vi "Find Data Replay Channels.vi"(6 "Custom Device Ref":T2 format="%.0x", 7 "Control String Info":T1, 8 "error in (no error)":errorcluster, 9 "Channel Descriptors in":T3, 11 "Replay ref":T2 format="%.0x") -> (0 "error out":errorcluster, 1 "Channel Descriptors out":T3)   [LabVIEW 2011, in "Engine Sim System Explorer.lvlib"]
uses:
  Engine Sim System Explorer.lvlib
  <vilib>/NI Veristand/Custom Device API/Custom Device Item Ref.ctl
  Shared/Channel Descriptors.ctl
  Shared/FPGA Write Descriptor.ctl
  Shared/InputChannelTypes.ctl
  <vilib>/rvi/DataTransferAndStorage/Container/Common/niFpgaDataTypeControl.ctl
  Shared/FPGA Read Descriptor.ctl
  Shared/OutputChannelTypes.ctl
  Shared/Status Chan Descriptor.ctl
  TypeDefs/DataReplayCtrlStringInfo.ctl
  Shared/Engine Simulation Global.vi
  <vilib>/NI Veristand/Custom Device Tools/Custom Device Utility Library/NI VeriStand - Search for Item by Name.vi
  <vilib>/NI Veristand/Custom Device Tools/Custom Device Utility Library/Custom Device Utility Library.lvlib
  Engine Simulation Shared.lvlib
  <vilib>/NI Veristand/Custom Device API/Custom Device API.lvlib
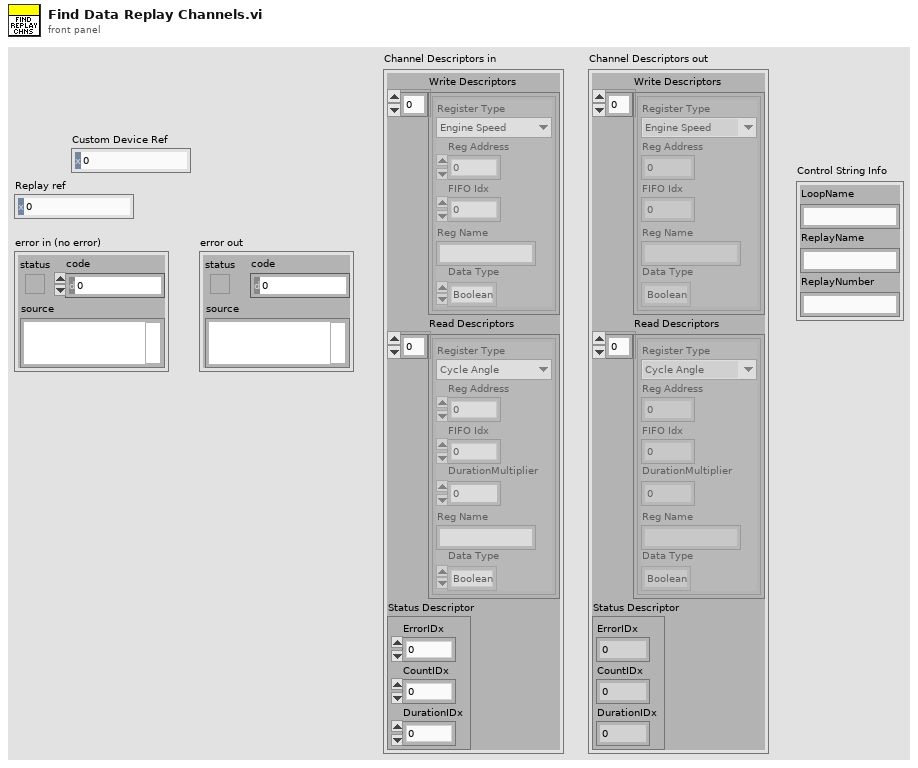
[diagram p1: front panel]
types:
  T1 = typedef "Engine Sim System Explorer.lvlib/DataReplayCtrlStringInfo.ctl" = cluster{"LoopName":string, "ReplayName":string, "ReplayNumber":string}
  T2 = typedef "Custom Device API.lvlib/Custom Device Item Ref.ctl" = u64
  T3 = typedef "Engine Simulation Shared.lvlib/Channel Descriptors.ctl" = cluster{"Write Descriptors":T4[], "Read Descriptors":T7[], "Status Descriptor":T9}
  T4 = typedef "Engine Simulation Shared.lvlib/FPGA Write Descriptor.ctl" = cluster{"Register Type":T5, "Reg Address":u32, "FIFO Idx":i32, "Reg Name":string, "Data Type":T6}
  T5 = typedef "Engine Simulation Shared.lvlib/InputChannelTypes.ctl" = enum16{"Engine Speed", "Offset"}
  T6 = typedef "niFpgaDataTypeControl.ctl" = enum32{"Boolean", "I8", "I16", "I32", "I64", "U8", "U16", "U32", "U64", "FXP", "CustomControl"}
  T7 = typedef "Engine Simulation Shared.lvlib/FPGA Read Descriptor.ctl" = cluster{"Register Type":T8, "Reg Address":u32, "FIFO Idx":i32, "DurationMultiplier":dbl, "Reg Name":string, "Data Type":T6}
  T8 = typedef "Engine Simulation Shared.lvlib/OutputChannelTypes.ctl" = enum16{"Cycle Angle", "Crank Angle", "Time Duration", "Angle Duration", "Start Angle", "End Angle"}
  T9 = typedef "Engine Simulation Shared.lvlib/Status Chan Descriptor.ctl" = cluster{"ErrorIDx":i32, "CountIDx":i32, "DurationIDx":i32}
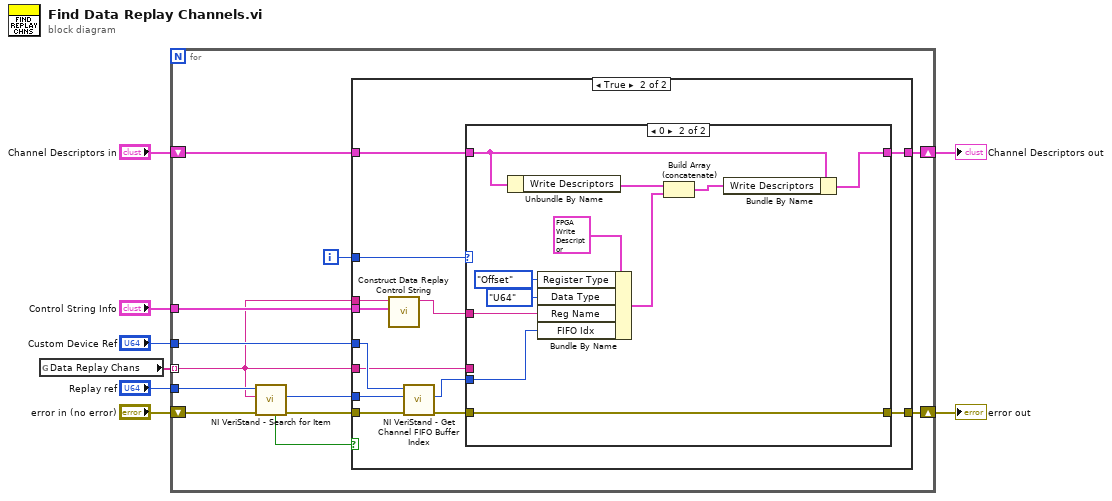
[diagram p0: block diagram]
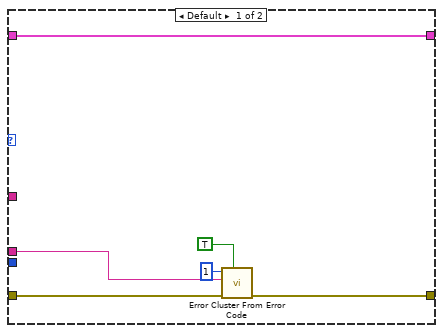
[diagram p3: hidden frame]
diagram:
  n1 = global read "Engine Simulation Global.vi" "Data Replay Chans"() -> (w4:string[])
  n2 = for {
    tunnel: "Replay ref" -> [w20]
    tunnel: "Custom Device Ref" -> [w14]
    shift-right: [w12] -> w5
    shift-left: "error in (no error)" -> [w19]
    shift-right: [w13] -> w6
    shift-left: "Channel Descriptors in" -> [w15]
    tunnel: w4 -> [w9] mode=indexing
    tunnel: "Control String Info" -> [w10]
    i -> [w11]
    n3 = call-poly <vilib>:"NI VeriStand - Search for Item.vi"("error in"=w19, "Item Name"=w9, "Section Ref in"=w20) -> ("error out"=w17:errorcluster, "Item Ref"=w16:T2, "Found"=w18:bool)  [unwired: 5 in, 1 out]
    n4 = case shown="True" w18 {
      tunnel: w17 -> [w21 w34]
      tunnel: w16 -> [_ w33]
      tunnel: w15 -> [w22 w35]
      tunnel: w14 -> [_ w32]
      tunnel: [w21 w27] -> w12
      tunnel: [w22 w30] -> w13
      tunnel: w11 -> [_ w29]
      tunnel: w10 -> [_ w26]
      tunnel: w9 -> [_ w25]
      tunnel: w9 -> [_ w23]
      frame False {
      }
      frame True {
        n5 = call "Construct Data Replay Control String.vi"("Control String Info"=w26, "Control Name"=w25) -> ("Control"=w24:string)  [unwired: 9 in]
        n6 = call <vilib>:"NI VeriStand - Get Channel FIFO Buffer Index.vi"("error in"=w34, "Channel Ref"=w33, "Device Ref in"=w32) -> ("error out"=w28:errorcluster, "Channel FIFO Buffer Index"=w31:i32)  [unwired: 4 in, 3 out]
        n7 = case shown="0" w29 {
          tunnel: w35 -> [w41 w51]
          tunnel: w31 -> [_ w49]
          tunnel: [w41 w47] -> w30
          tunnel: w24 -> [_ w45]
          tunnel: w28 -> [w40 w43]
          tunnel: [w39 w43] -> w27
          tunnel: w23 -> [w36 _]
          frame Default {
            n8 = call <vilib>:"Error Cluster From Error Code.vi"("show call chain? (False)"=TRUE, "error in (no error)"=w40, "error message (\"\")"=w36, "error code (0)"=1) -> ("error out"=w39:errorcluster)  [unwired: 5 in]
          }
          frame 0 {
            n9 = Unbundle By Name(w51) -> ("Write Descriptors"=w52:T4[])
            n10 = Bundle By Name(cluster=T4 {"Register Type"=enum."Engine Speed", "Reg Address"=0, "FIFO Idx"=0, "Reg Name"="", "Data Type"=enum."Boolean"} ("Write Descriptor"), "Register Type"=InputChannelTypes."Offset", "Data Type"=niFpgaDataTypeControl."U64", "Reg Name"=w45, "FIFO Idx"=w49) -> (w46:T4)
            n11 = Build Array (concatenate)(w52, w46) -> (w48:T4[])
            n12 = Bundle By Name(cluster=w51, "Write Descriptors"=w48) -> (w47:T3)
          }
        }
      }
    }
  }
  "error out" <- w5
  "Channel Descriptors out" <- w6
